vi "Fire DAQStateChanged Event_DAQ.vi"(8 "error in (no error)":errorcluster, 9 "vData":variant, 10 "DAQState":variant, 11 "DAQ_Engine in":refnum<class "DAQ_Engine.lvclass">) -> (0 "error out":errorcluster, 3 "DAQ_Engine out":refnum<class "DAQ_Engine.lvclass">)   [LabVIEW 2019, in "DAQ_Engine.lvclass"]
doc: "Developed by Kevin Thompson\nkevin@thompsonengineering.net\n\nCopyright 2018-2020\nThompson Engineering, LLC"
uses:
  DAQ_Engine.lvclass
  Common/DataTypes/DAQState--enum.ctl
  DataTypes/DAQStateEvData--cluster.ctl
  DataTypes/DAQStateChg EvData--cluster.ctl
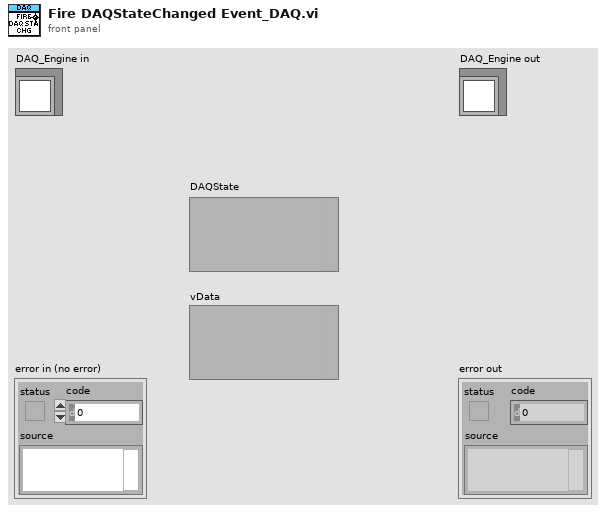
[diagram p1: front panel]
types:
  T1 = typedef "DAQ_Engine.lvclass/DAQStateChg EvData--cluster.ctl" = cluster{"Time Stamp":timestamp, "OLD State":T2, "NEW State":T2}
  T2 = typedef "DAQ_Engine.lvclass/DAQStateEvData--cluster.ctl" = cluster{"DAQState":T3, "vData":variant}
  T3 = typedef "DAQState--enum.ctl" = enum16{"Unknown", "Stopped", "Running", "Error"}
  T4 = typedef "DAQ_Engine.lvclass/Public Events--cluster.ctl" = cluster{"DAQ_Engine.AsyncCmd Event":refnum<user-event>, "DAQ_Engine.AsyncMsg Event":refnum<user-event>, "stop process":refnum<user-event>, "DAQ_Engine.DAQStateChg Ev":refnum<user-event>, "DAQ_Engine.MeasSettingsChg Ev":refnum<user-event>, "DAQ_Engine.AcqModeChg Ev":refnum<user-event>}
  T5 = typedef "DAQStateEvData--cluster.ctl" = cluster{"DAQState":T3, "vData":variant}
  T6 = typedef "Type Descriptor Enumeration__ogtk.ctl" = enum8{"<Null>", "I8", "I16", "I32", "I64", "U8", "U16", "U32", "U64", "SGL", "DBL", "EXT", "CSG", "CDB", "CXT", "0x0F", "0x10", "0x11", "0x12", "0x13", "0x14", "Enum U8", "Enum U16", "Enum U32", "Enum U64", "SGL PQ", "DBL PQ", "EXT PQ", "CSG PQ", "CDB PQ", "CXT PQ", "0x1F", "0x20", "Boolean", "0x22", "0x23", "0x24", "0x25", "0x26", "0x27", "0x28", "0x29", "0x2A", "0x2B", "0x2C", "0x2D", "0x2E", "0x2F", "String", "0x31", "Path", "Pict", "0x34", "0x35", "0x36", "DAQ", "0x38", "0x39", "0x3A", "0x3B", "0x3C", "0x3D", "0x3E", "0x3F", "Array", "0x41", "0x42", "0x43", "0x44", "0x45", "0x46", "0x47", "0x48", "0x49", "0x4A", "0x4B", "0x4C", "0x4D", "0x4E", "0x4F", "Cluster", "0x51", "0x52", "Variant", "Waveform", "0x55", "0x56", "0x57", "0x58", "0x59", "0x5A", "0x5B", "0x5C", "0x5D", "0x5E", "0x5F", "0x60", "0x61", "0x62", "0x63", "0x64", "0x65", "0x66", "0x67", "0x68", "0x69", "0x6A", "0x6B", "0x6C", "0x6D", "0x6E", "0x6F", "Refnum"}
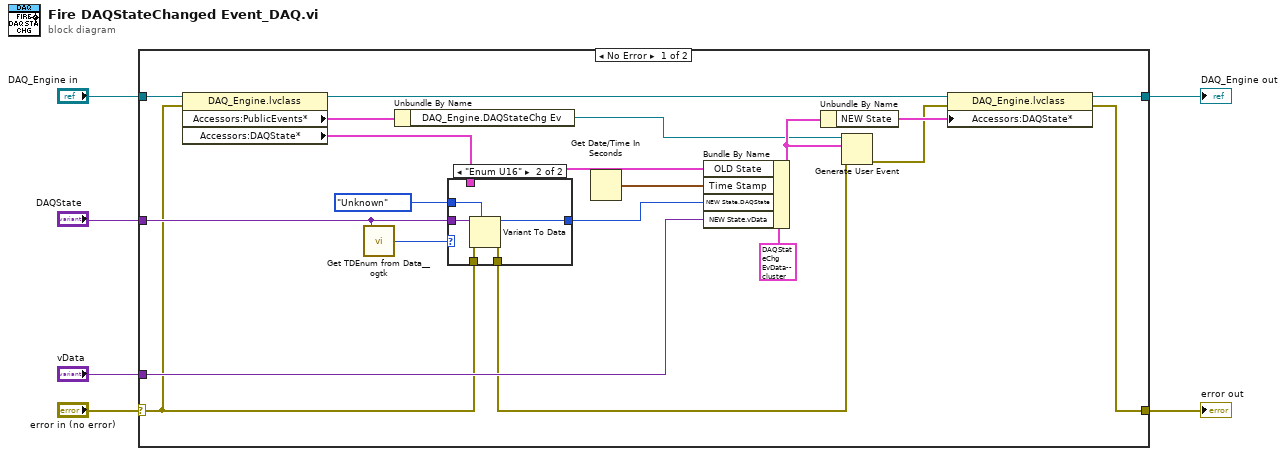
[diagram p0: block diagram]
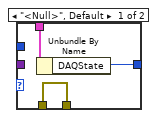
[diagram p2: hidden frame]
diagram:
  n1 = case shown="No Error" "error in (no error)" {
    selector: "error in (no error)" -> [w12 w35]
    tunnel: [w13 w35] -> w5
    tunnel: [w17 w34] -> w3
    tunnel: "DAQ_Engine in" -> [w24 w34]
    tunnel: "DAQState" -> [w22 _]
    tunnel: "vData" -> [w19 _]
    frame No Error {
      n2 = property class="DAQ_Engine.lvclass"(reference=w24, error in=w12) -> (reference out=w7:refnum<class "DAQ_Engine.lvclass">, "Accessors:PublicEvents*"=w8:T4, "Accessors:DAQState*"=w9:T5)  [unwired: 1 out]
      n3 = call <userlib>:"Get TDEnum from Data__ogtk.vi"("Data"=w22) -> ("Type Descriptor Enumeration"=w23:T6)  [unwired: 4 in]
      n4 = Unbundle By Name(w8) -> ("DAQ_Engine.DAQStateChg Ev"=w10:refnum<user-event>)
      n5 = case shown="\"Enum U16\"" w23 {
        tunnel: w9 -> [w28 _]
        tunnel: w22 -> [_ w33]
        tunnel: [w27 w32] -> w20
        tunnel: DAQState--enum."Unknown" ("DAQState") -> [_ w31]
        tunnel: w12 -> [w26 w30]
        tunnel: [w26 w29] -> w18
        frame "<Null>", Default {
          n6 = Unbundle By Name(w28) -> ("DAQState"=w27:T3)
        }
        frame "Enum U16" {
          n7 = Variant To Data(error in=w30, type=w31, Variant=w33) -> (data=w32:T3, error out=w29:errorcluster)
        }
      }
      n8 = Get Date/Time In Seconds() -> (seconds since 1Jan1904=w25:timestamp)
      n9 = Bundle By Name(cluster=T1 {"Time Stamp"=timestamp(0 s since 1904-01-01), "OLD State"={"DAQState"=enum."Unknown", "vData"=variant}, "NEW State"={"DAQState"=enum."Unknown", "vData"=variant}} ("DAQStateChanged EventData"), "OLD State"=w9, "Time Stamp"=w25, "NEW State.DAQState"=w20, "NEW State.vData"=w19) -> (w16:T1)
      n10 = Unbundle By Name(w16) -> ("NEW State"=w15:T2)
      n11 = Generate User Event(user event=w10, event data cluster=w16, error in=w18) -> (error out=w14:errorcluster)  [unwired: 1 in, 1 out]
      n12 = property class="DAQ_Engine.lvclass"(reference=w7, error in=w14, "Accessors:DAQState*"=w15) -> (reference out=w17:refnum<class "DAQ_Engine.lvclass">, error out=w13:errorcluster)
    }
    frame Error {
    }
  }
  "error out" <- w5
  "DAQ_Engine out" <- w3
